vi "Copy .LLB to NI VeriStand dir.vi"(5 "Files Generated by Build":path[](array[path]), 6 "Top Level/Always Included VIs":path[](array[path]), 7 "Destination Path":path, 8 "error in (no error)":errorcluster, 9 "Target Name":string, 10 "Build Specification Name":string, 11 "Project Path":path) -> (0 "error out":errorcluster)   [LabVIEW 2024]
doc: "This VI is called after each run of a build specification. The VI will copy the generated LLB (Engine or System Explorer) into the VeriStand Custom Device folder (...\\Documents\\National Instruments\\NI VeriStand 2013...)."
uses:
  C:/Users/ppathak/Downloads/NationalInstruments.VeriStand.dll
  Users/ppathak/Downloads/NationalInstruments.VeriStand.dll
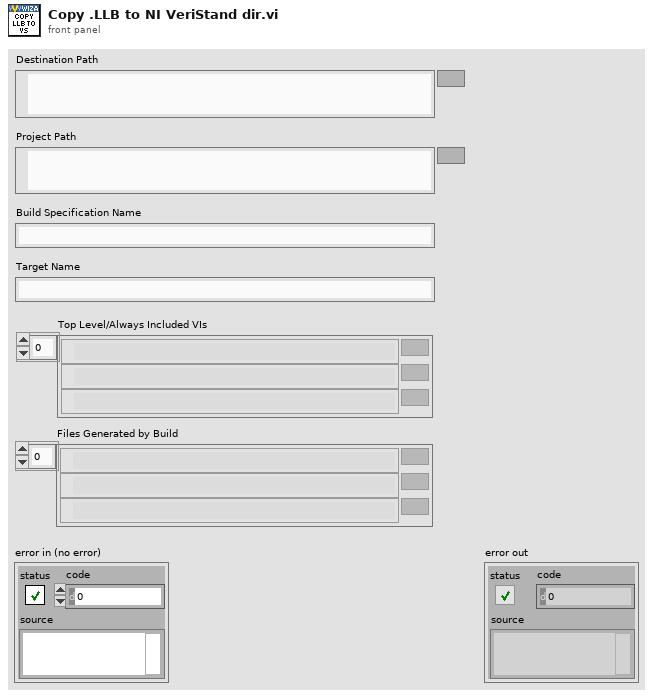
[diagram p1: front panel]
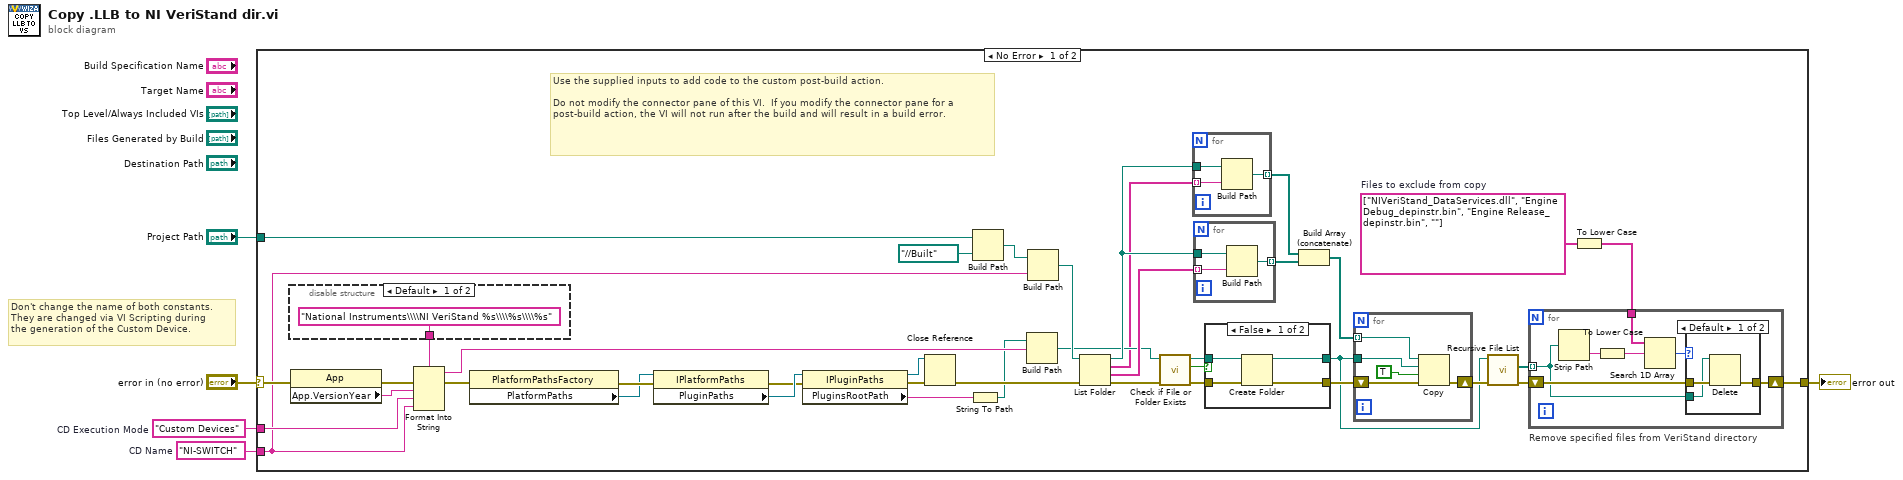
[diagram p0: block diagram]
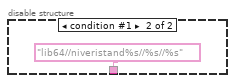
[diagram p2: hidden frame]
diagram:
  w2 = "NI-SWITCH"  # CD Name
  w3 = "Custom Devices"  # CD Execution Mode
  # "Don't change the name of both constants.\nThey are changed via VI Scripting during\nthe generation of the Custom Device."
  n1 = case shown="No Error" "error in (no error)" {
    selector: "error in (no error)" -> [w30 w76]
    tunnel: [w18 w76] -> w1
    tunnel: "Project Path" -> [w27 _]
    tunnel: w3 -> [w31 _]
    tunnel: w2 -> [w29 _]
    frame No Error {
      w24 = string[] ["NIVeriStand_DataServices.dll", "Engine Debug_depinstr.bin", "Engine Release_depinstr.bin", ""]  # Files to exclude from copy
      # "Use the supplied inputs to add code to the custom post-build action.\n\nDo not modify the connector pane of this VI.  If you modify the connector pane for a post-build action, the VI will not run after the build and will result in a build error."
      n2 = disable-structure shown="Default" {
        disable-tunnel: ["National Instruments\\\\NI VeriStand %s\\\\%s\\\\%s" ("name or relative path") "lib64//niveristand%s//%s//%s" ("name or relative path")] -> w33
        frame condition #0 (active) {
        }
        frame condition #1 {
        }
      }
      n3 = property class="App"(error in=w30) -> (error out=w35:errorcluster, "App.VersionYear"=w34:string)  [unwired: 1 in, 1 out]
      n4 = Format Into String(format string=w33, error in=w35, w34, w31, w29) -> (resulting string=w16:string, error out=w7:errorcluster)  [unwired: 1 in]
      n5 = property class="PlatformPathsFactory"(error in=w7) -> (error out=w14:errorcluster, "PlatformPaths"=w12:refnum<k24>)  [unwired: 1 in, 1 out]
      n6 = property class="IPlatformPaths"(reference=w12, error in=w14) -> (error out=w13:errorcluster, "PluginPaths"=w15:refnum<k24>)  [unwired: 1 out]
      n7 = property class="IPluginPaths"(reference=w15, error in=w13) -> (reference out=w6:refnum<k24>, error out=w10:errorcluster, "PluginsRootPath"=w11:string)
      n8 = Close Reference(reference=w6, error in (no error)=w10) -> (error out=w9:errorcluster)
      n9 = String To Path(string=w11) -> (path=w8:path)
      n10 = Build Path(base path=w27, name or relative path=path "../../Built") -> (appended path=w17:path)
      n11 = Build Path(base path=w8, name or relative path=w16) -> (appended path=w32:path)
      n12 = Build Path(base path=w17, name or relative path=w29) -> (appended path=w37:path)
      n13 = List Folder(path=w37, error in=w9) -> (path out=w39:path, filenames=w25:string[], folder names=w40:string[], error out=w36:errorcluster)  [unwired: 2 in]
      n14 = call <vilib>:"Check if File or Folder Exists.vi"("error in (no error)"=w36, "path"=w32) -> ("error out"=w41:errorcluster, "file or folder exists?"=w43:bool, "dup path"=w42:path)  [unwired: 7 in]
      n15 = for {
        tunnel: w25 -> [w74] mode=indexing
        tunnel: w39 -> [w75]
        tunnel: [w73] -> w45 mode=indexing
        n16 = Build Path(base path=w75, name or relative path=w74) -> (appended path=w73:path)
      }
      n17 = for {
        tunnel: w40 -> [w71] mode=indexing
        tunnel: w39 -> [w72]
        tunnel: [w70] -> w38 mode=indexing
        n18 = Build Path(base path=w72, name or relative path=w71) -> (appended path=w70:path)
      }
      n19 = case shown="False" w43 {
        tunnel: w42 -> [w62 w64]
        tunnel: w41 -> [w61 w63]
        tunnel: [w60 w64] -> w19
        tunnel: [w59 w63] -> w26
        frame False {
          n20 = Create Folder(path (use dialog)=w62, error in=w61) -> (created path=w60:path, error out=w59:errorcluster)  [unwired: 1 in, 1 out]
        }
        frame True {
        }
      }
      n21 = Build Array (concatenate)(w45, w38) -> (w44:path[])
      n22 = for {
        tunnel: w44 -> [w66] mode=indexing
        shift-right: [w67] -> w20
        shift-left: w26 -> [w68]
        tunnel: w19 -> [w65]
        n23 = Copy(8:w68, 9:TRUE ("overwrite (F)"), 10:w65, 11:w66) -> (0:w67:errorcluster)  [unwired: 1 in, 2 out]
      }
      n24 = call <vilib>:"Recursive File List.vi"("error in (no error)"=w20, "Folder Path"=w19) -> ("error out"=w23:errorcluster, "All Files in Dir"=w22:path[])  [unwired: 5 in, 3 out]
      n25 = To Lower Case(string=w24) -> (all lower case string=w21:string[])
      n26 = for "Remove specified files from VeriStand directory" {
        shift-right: [w49] -> w18
        shift-left: w23 -> [w51]
        tunnel: w22 -> [w48] mode=indexing
        tunnel: w21 -> [w52]
        n27 = Strip Path(path=w48) -> (name=w54:string)  [unwired: 1 out]
        n28 = To Lower Case(string=w54) -> (all lower case string=w53:string)
        n29 = Search 1D Array(1D array=w52, element=w53) -> (index of element=w50:i32)  [unwired: 1 in]
        n30 = case shown="Default" w50 {
          tunnel: w51 -> [w57 w58]
          tunnel: [w56 w58] -> w49
          tunnel: w48 -> [w55 _]
          frame Default {
            n31 = Delete(path (use dialog)=w55, error in=w57) -> (error out=w56:errorcluster)  [unwired: 3 in, 2 out]
          }
          frame -1 {
          }
        }
      }
    }
    frame Error {
    }
  }
  "error out" <- w1
